vi "Create Handlers from Config.vi"(8 "error in (no error)":errorcluster, 11 "DataProcessor in":refnum<class "DataProcessor.lvclass">) -> (0 "error out":errorcluster, 3 "DataProcessor out":refnum<class "DataProcessor.lvclass">)   [LabVIEW 2020, in "VolatusData.lvlib" / "DataProcessor.lvclass"]
uses:
  DataProcessor.lvclass
  DataProcessor.lvclass/DataProcessor.ctl
  Volatus/Task/Task.lvclass
  lv-cdm/CDM-Config/Config Element/Config Element.lvclass
  Volatus/Volatus.lvlib
  C:/dev/lv20CE/relink/lv-volatus/VolatusData/DataHandlerTask/DataHandlerTask.lvclass
  C:/dev/lv20CE/relink/lv-volatus/Volatus/Task/Task.lvclass
  C:/Program Files (x86)/National Instruments/LabVIEW 2020/vi.lib/ActorFramework/Actor/Actor.lvclass
  C:/dev/lv20CE/relink/lv-volatus/Volatus/TaskStateHandler/TaskStateHandler.lvclass
  C:/dev/lv20CE/relink/lv-volatus/Volatus/VectoMessageHandler/VectoMessageHandler.lvclass
  C:/dev/lv20CE/relink/lv-volatus/Volatus/API Provider/API Provider.lvclass
  C:/dev/lv20CE/relink/lv-volatus/VolatusData/DataHandler/DataHandler.lvclass
  C:/dev/lv20CE/relink/lv-volatus/VolatusData/DataProcessor/DataProcessor.lvclass
  C:/dev/lv20CE/relink/lv-volatus/Volatus/Abortable/Abortable.lvclass
  C:/dev/lv20CE/relink/lv-volatus/Volatus/Reconfigurable/Reconfigurable.lvclass
  DataHandlerAPI/DataHandlerAPI.lvclass
  VolatusConfig/VolatusConfigElement/VolatusConfigElement.lvclass
  VolatusConfig/Task/Task.lvclass
  C:/dev/lv20CE/relink/lv-volatus/VolatusConfig/VolatusConfigElement/VolatusConfigElement.lvclass
  C:/dev/lv20CE/relink/lv-volatus/VolatusConfig/Task/Task.lvclass
  C:/dev/lv20CE/relink/lv-volatus/VolatusData/DataHandlerAPI/DataHandlerAPI.lvclass
  C:/dev/lv20CE/relink/lv-volatus/Volatus/API/API.lvclass
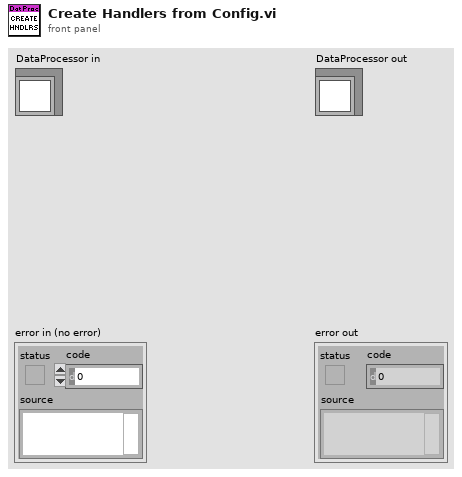
[diagram p1: front panel]
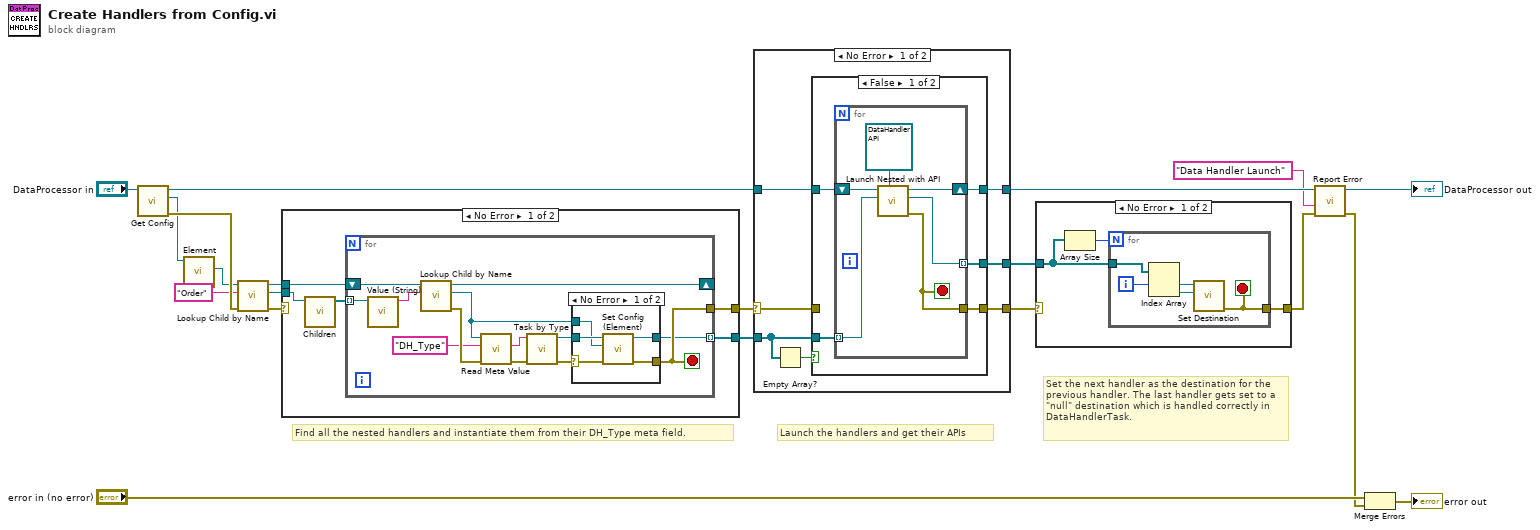
[diagram p0: block diagram]
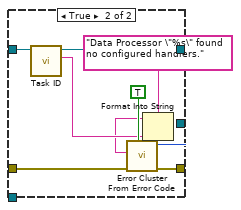
[diagram p5: hidden frame]
diagram:
  # "Set the next handler as the destination for the previous handler. The last handler gets set to a \"null\" destination which is handled correctly in DataHandlerTask."
  # "Launch the handlers and get their APIs"
  # "Find all the nested handlers and instantiate them from their DH_Type meta field."
  n1 = call "Get Config.vi"("Task in"="DataProcessor in") -> ("error out"=w20:errorcluster, "Config"=w17:refnum<class "Task.lvclass">, "Task out"=w9:refnum<class "DataProcessor.lvclass">)  [unwired: 8 in]
  n2 = call "Element.vi"("VolatusConfigElement in"=w17) -> ("Element"=w16:refnum<class "Config Element.lvclass">)  [unwired: 9 in, 1 out]
  n3 = call "Lookup Child by Name.vi"("error in (no error)"=w20, "Name"="Order", "Config Element in"=w16) -> ("error out"=w12:errorcluster, "Child"=w14:refnum<class "Config Element.lvclass">, "Config Element out"=w13:refnum<class "Config Element.lvclass">)  [unwired: 5 in, 1 out]
  n4 = case shown="No Error" w12 {
    selector: w12 -> [_ w45]
    tunnel: w14 -> [w25 _]
    tunnel: w13 -> [w23 _]
    tunnel: [w22 w45] -> w11
    tunnel: [w21 _] -> w10
    frame No Error {
      n5 = call "Children.vi"("Config Element in"=w25) -> ("Elements"=w24:refnum<class "Config Element.lvclass">[])  [unwired: 9 in, 1 out]
      n6 = for {
        tunnel: w24 -> [w37] mode=indexing
        shift-right: [w34] -> _
        shift-left: w23 -> [w36]
        tunnel: [w38] -> w22
        tunnel: [w26] -> w21 mode=indexing
        stop <- w38 stop-if-true
        n7 = call "Value (String).vi"("Config Element in"=w37) -> ("String Value"=w35:string)  [unwired: 9 in, 1 out]
        n8 = call "Lookup Child by Name.vi"("Name"=w35, "Config Element in"=w36) -> ("error out"=w33:errorcluster, "Child"=w27:refnum<class "Config Element.lvclass">, "Config Element out"=w34:refnum<class "Config Element.lvclass">)  [unwired: 6 in, 1 out]
        n9 = call "Read Meta Value.vi"("error in (no error)"=w33, "Meta Name"="DH_Type", "Config Element in"=w27) -> ("error out"=w31:errorcluster, "Meta Value"=w30:string)  [unwired: 6 in, 1 out]
        n10 = call "Task by Type.vi"("error in (no error)"=w31, "Task Type"=w30) -> ("error out"=w28:errorcluster, "Task"=w29:refnum<class "Task.lvclass">)  [unwired: 8 in]
        n11 = case shown="No Error" w28 {
          selector: w28 -> [w42 w44]
          tunnel: w29 -> [w43 _]
          tunnel: w27 -> [w41 _]
          tunnel: [w40 _] -> w26
          tunnel: [w39 w44] -> w38
          frame No Error {
            n12 = call "Set Config (Element).vi"("error in (no error)"=w42, "Config Element"=w41, "Task in"=w43) -> ("error out"=w39:errorcluster, "Task out"=w40:refnum<class "Task.lvclass">)  [unwired: 7 in]
          }
          frame Error {
          }
        }
      }
    }
    frame Error {
    }
  }
  n13 = case shown="No Error" w11 {
    selector: w11 -> [w48 w74]
    tunnel: w10 -> [w50 _]
    tunnel: w9 -> [w52 w73]
    tunnel: [w51 w73] -> w8
    tunnel: [w47 w74] -> w6
    tunnel: [w46 _] -> w7
    frame No Error {
      n14 = Empty Array?(array=w50) -> (empty?=w49:bool)
      n15 = case shown="False" w49 {
        tunnel: w50 -> [w55 _]
        tunnel: w52 -> [w57 w69]
        tunnel: [w56 w66] -> w51
        tunnel: w48 -> [_ w65]
        tunnel: [w54 w64] -> w47
        tunnel: [w53 _] -> w46
        frame False {
          n16 = for {
            shift-right: [w60] -> w56
            shift-left: w57 -> [w63]
            tunnel: w55 -> [w62] mode=indexing
            tunnel: [w59] -> w53 mode=indexing
            tunnel: [w58] -> w54
            stop <- w58 stop-if-true
            n17 = call "Launch Nested with API.vi"("API Type"=refnum<class "DataHandlerAPI.lvclass"> refnum ("Volatus:DataHandlerAPI"), "Nested Task"=w62, "Task in"=w63) -> ("error out"=w58:errorcluster, "API"=w59:refnum<class "DataHandlerAPI.lvclass">, "Task out"=w60:refnum<class "DataProcessor.lvclass">)  [unwired: 6 in]
          }
        }
        frame True {
          n18 = call-dynamic "Task ID.vi"("DataProcessor in"=w69) -> ("Task ID"=w68:string, "DataProcessor out"=w66:refnum<class "DataProcessor.lvclass">)  [unwired: 8 in, 1 out]
          n19 = Format Into String(format string="Data Processor \"%s\" found no configured handlers.", w68) -> (resulting string=w67:string)  [unwired: 2 in, 1 out]
          n20 = call <vilib>:"Error Cluster From Error Code.vi"("show call chain? (False)"=TRUE, "error in (no error)"=w65, "error message (\"\")"=w67, "error code (0)"=15) -> ("error out"=w64:errorcluster)  [unwired: 5 in]
        }
      }
    }
    frame Error {
    }
  }
  n21 = case shown="No Error" w6 {
    selector: w6 -> [_ w83]
    tunnel: w7 -> [w76 _]
    tunnel: [w75 w83] -> w4
    frame No Error {
      n22 = Array Size(array=w76) -> (size(s)=w77:i32)
      n23 = for {
        N: w77 -> [_]
        tunnel: w76 -> [w82]
        tunnel: [w78] -> w75
        i -> [w81]
        stop <- w78 stop-if-true
        n24 = Index Array(array=w82, index #1=w81) -> (element #1=w80:refnum<class "DataHandlerAPI.lvclass">, element #2=w79:refnum<class "DataHandlerAPI.lvclass">)  [unwired: 1 in]
        n25 = call-dynamic "Set Destination.vi"("Destination"=w79, "DataHandlerAPI in"=w80) -> ("error out"=w78:errorcluster)  [unwired: 8 in, 1 out]
      }
    }
    frame Error {
    }
  }
  n26 = call "Report Error.vi"("error in (no error)"=w4, "Message"="Data Handler Launch", "Task in"=w8) -> ("error out"=w1:errorcluster, "Task out"=→"DataProcessor out":refnum<class "DataProcessor.lvclass">)  [unwired: 7 in]
  n27 = Merge Errors("error in (no error)", w1) -> (→"error out":errorcluster)
